vi "Syringe Pump Controller.vi"() -> ()   [LabVIEW 2012]
uses:
  Type/_Syringe Pump Command.ctl
  Type/_RT Serial Command.ctl
  Type/_RT Command.ctl
panel:
  in  "Send":bool
  out "Raw Reply":string
  out "Telegram":string
  in  "Input Value":sgl
  in  "Pump Command":T1
  # "For the RS232-1 serial chanel supported through FPGA using pins:\nPort5.0 for RXD and 5.1 for TXD"
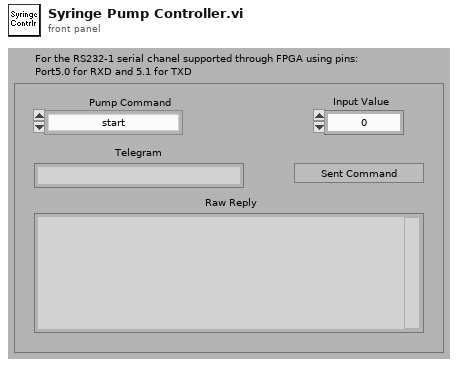
[diagram p1: front panel]
types:
  T1 = typedef "_Syringe Pump Command.ctl" = enum16{"start", "stop", "pause", "restart", "help", "set units", "set diameter", "set rate", "set time", "set volume", "set delay", "save setting", "read limit parameter", "view parameter", "status"}
  T2 = typedef "_RT Serial Command.ctl" = cluster{"Port Type":u16, "baud rate (9600)":u32, "data bits (8)":u16, "stop bits (1)":u16, "parity (0:none)":u16, "DoRead":bool, "Command":string}
  T3 = typedef "_RT Command.ctl" = enum16{"Start", "Stop", "Runtime Update", "Get Data", "Get Info", "Get Status", "Get Param", "Get Config", "Get Table", "Read ADC", "Set Oscillator", "Update Config", "Update Table", "Set All Pol", "Set Pol and DC", "Set Max Mass", "Toggle RP", "Toggle EL", "Set PIC", "Initialize Turbo", "Send Turbo Comm", "Close Turbo", "P1", "P2", "P3", "Send Serial", "Set LC Out", "Get LC In", "Read VAC", "Test Table", "Toggle Power", "Get Startup", "Set Startup", "Get ADC Table", "Set ADC Table", "Get Brief Status", "Get Detail Status", "Auxiliary Update", "Set CC Logics", "Set CC Input Logics", "Ignore Error"}
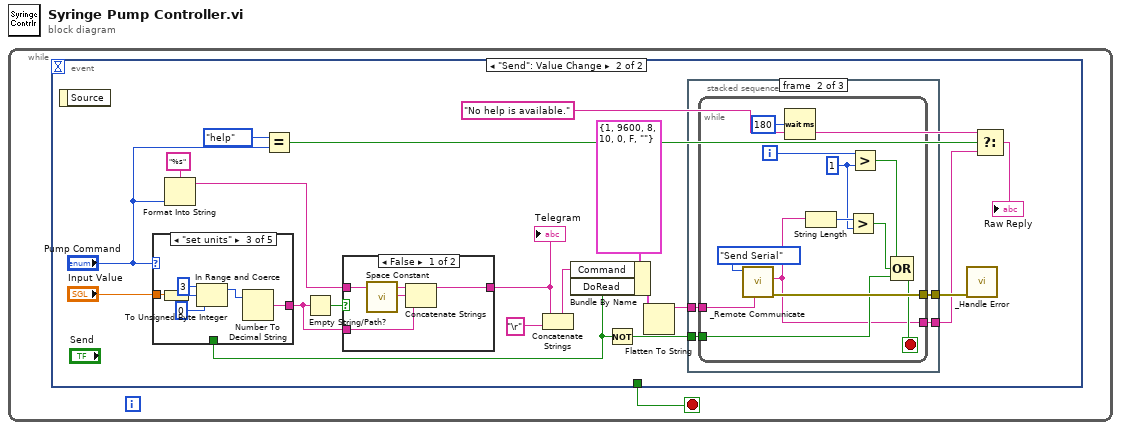
[diagram p0: block diagram]
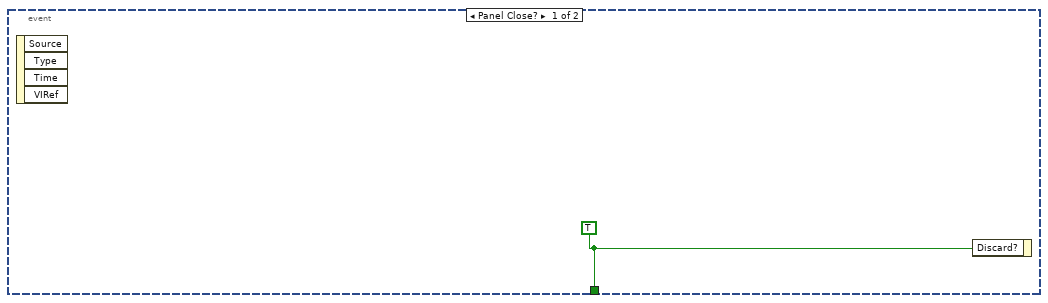
[diagram p2: hidden frame]
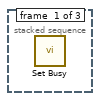
[diagram p3: hidden frame]
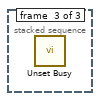
[diagram p4: hidden frame]
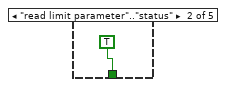
[diagram p6: hidden frame]
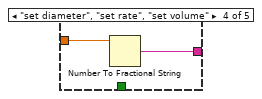
[diagram p7: hidden frame]
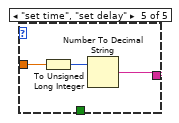
[diagram p8: hidden frame]
diagram:
  n1 = while {
    stop <- w1 stop-if-true
    n2 = event shown="[1] \"Send\": Value Change" {
      selector: _ -> [_ _]
      dyn-events: _ -> [_ _]
      timeout: _ -> [_ _]
      tunnel: [w2 _] -> w1
      event Panel Close? {
        w2 = TRUE
        n3 = event-data() -> ()  [unwired: 5 out]
        n4 = event-data("Discard?"=w2) -> ()  [unwired: 1 in, 1 out]
      }
      event "Send": Value Change {
        n5 = event-data() -> ()  [unwired: 2 out]
        n6 = case shown="\"set units\"" "Pump Command" {
          tunnel: "Input Value" -> [_ _ w45 w47 w49]
          tunnel: [_ _ w43 w46 w48] -> w11
          tunnel: [_ TRUE _ _ _] -> w10
          frame Default {
          }
          frame "read limit parameter".."status" {
          }
          frame "set units" {
            n7 = To Unsigned Byte Integer(number=w45) -> (unsigned 8bit integer=w44:u8)
            n8 = In Range and Coerce(upper limit=u8 3, x=w44, lower limit=u8 0) -> (coerced(x)=w42:u8)  [unwired: 1 out]
            n9 = Number To Decimal String(number=w42) -> (decimal integer string=w43:string)  [unwired: 1 out]
          }
          frame "set diameter", "set rate", "set volume" {
            n10 = Number To Fractional String(number=w47) -> (F-format string=w46:string)  [unwired: 3 out]
          }
          frame "set time", "set delay" {
            n11 = To Unsigned Long Integer(number=w49) -> (unsigned 32bit integer=w50:u32)
            n12 = Number To Decimal String(number=w50) -> (decimal integer string=w48:string)  [unwired: 1 out]
          }
        }
        n13 = Format Into String(format string="%s", "Pump Command") -> (resulting string=w14:string)  [unwired: 2 in, 1 out]
        n14 = Equal?(x=_Syringe_Pump_Command."help", y="Pump Command") -> (x = y?=w6:bool)
        n15 = Empty String/Path?(string/path=w11) -> (empty?=w15:bool)
        n16 = case shown="False" w15 {
          tunnel: w11 -> [w52 _]
          tunnel: w14 -> [w54 w55]
          tunnel: [w51 w55] -> w13
          frame False {
            n17 = call <vilib>:"Space Constant.vi"() -> ("String"=w53:string)
            n18 = Concatenate Strings(w54, w53, w52) -> (w51:string)
          }
          frame True {
          }
        }
        "Telegram" <- w13
        n19 = Concatenate Strings(w13, "\r" ("string")) -> (w18:string)
        n20 = Bundle By Name(cluster=T2 {"Port Type"=1, "baud rate (9600)"=9600, "data bits (8)"=8, "stop bits (1)"=10, "parity (0:none)"=0, "DoRead"=FALSE, "Command"=""} ("Serial Command"), "Command"=w18, "DoRead"=w10) -> (w17:T2)
        n21 = Not(x=w10) -> (.not. x?=w9:bool)
        n22 = Flatten To String(anything=w17) -> (data string=w22:string)  [unwired: 1 in, 4 out]
        n23 = stacked-sequence {
          tunnel: w22 -> [_ w26 _]
          tunnel: [_ w25 _] -> w21
          tunnel: [_ w24 _] -> w5
          tunnel: w9 -> [_ w23 _]
          frame #0 {
            n24 = call <vilib>:"Set Busy.vi"() -> ()  [unwired: 4 in, 8 out]
          }
          frame #1 {
            n25 = while {
              tunnel: w26 -> [w38]
              tunnel: [w36] -> w25
              tunnel: [w30] -> w24
              tunnel: w23 -> [w32]
              i -> [w35]
              stop <- w31 stop-if-true
              w28 = 1 ("y")
              n26 = call "_Remote Communicate.vi"("String"=w38, "Command"=_RT_Command."Send Serial") -> ("error out"=w36:errorcluster, "Info"=w30:string)  [unwired: 4 in, 2 out]
              n27 = Wait (ms)(milliseconds to wait=u32 180) -> ()  [unwired: 1 out]
              n28 = String Length(string=w30) -> (length=w29:i32)
              n29 = Greater?(x=w29, y=w28) -> (0:w27:bool)
              n30 = Greater?(x=w35, y=w28) -> (0:w33:bool)
              n31 = Compound Arithmetic op=OR(w33, w27, w32) -> (w31:bool)
            }
          }
          frame #2 {
            n32 = call <vilib>:"Unset Busy.vi"() -> ()  [unwired: 2 in, 10 out]
          }
        }
        n33 = call "_Handle Error.vi"("error in (no error)"=w21) -> ()  [unwired: 2 in, 5 out]
        n34 = Select(t="No help is available.", s=w6, f=w5) -> (s? t:f=→"Raw Reply":string)
      }
    }
  }
